vi "rspvtd_Connection Lost.vi"(8 "error in":errorcluster, 11 "Data in":variant) -> (0 "error out":errorcluster, 3 "Data out":T1)   [LabVIEW 2017, in "DS TCP Server.lvlib" / "DS TCP Read.lvclass"]
doc: "This VI converts variant data contained in the associated <b>Public API Response</b> message to its correct data type.\n---"
uses:
  DS TCP Read.lvclass
  rsp_Connection Lost.ctl
  <vilib>/addons/_Workers/Library/Classes/Message Queue/Message Queue.lvclass
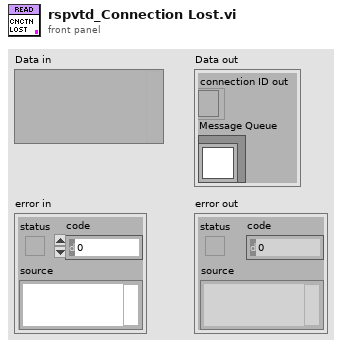
[diagram p1: front panel]
types:
  T1 = typedef "DS TCP Server.lvlib/DS TCP Read.lvclass/rsp_Connection Lost.ctl" = cluster{"connection ID out":refnum<k5>, "Message Queue":refnum<class "Message Queue.lvclass">}
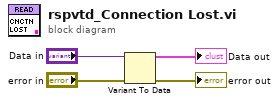
[diagram p0: block diagram]
diagram:
  n1 = Variant To Data(error in="error in", Variant="Data in") -> (data=→"Data out":T1, error out=→"error out":errorcluster)  [unwired: 1 in]
